vi "BT Example 1 - Repeater.vi"() -> ()   [LabVIEW 2021]
uses:
  Support/Nodes/abs_Node/Status.ctl
  Blackboard/Blackboard.lvclass
  Support/Nodes/Decorators/Repeater/Support/Finish On - Type.ctl
  System/bt_System.lvclass
  Blackboard/Blackboard.lvclass/Blackboard.ctl
  Blackboard/Get Value Type/Get I32.vi
  Blackboard/Support/Index Group.vi
  Blackboard/Support/Index Tags.vi
  <vilib>/TSA/Omni-Bus/Local Bus/Support/I32/Local Bus_I32.lvclass
  C:/Program Files (x86)/National Instruments/LabVIEW 2021/vi.lib/TSA/Abstract Data Classes/Abs_Types/Value/Abs_Value.lvclass
  <vilib>/TSA/Abstract Data Classes/Abs_Types/I32 Integer/Abs_I32 Integer.lvclass
  <vilib>/TSA/Omni-Bus/Local Bus/Support/Initialise DVR's.vi
  <vilib>/TSA/Abstract Data Classes/Functions/Math/Support/Increment/I32/Method.vi
  <vilib>/TSA/Abstract Data Classes/Abs_Types/Value/Abs_Value.lvclass
  <vilib>/TSA/Abstract Data Classes/Abs_Types/Type/Abs_Type.lvclass
  <vilib>/TSA/Omni-Bus/Local Bus/Support/DBL/Local Bus_DBL.lvclass
  <vilib>/TSA/Omni-Bus/Local Bus/Support/SGL/Local Bus_SGL.lvclass
  <vilib>/TSA/Omni-Bus/Local Bus/Support/EXT/Local Bus_EXT.lvclass
  <vilib>/TSA/Omni-Bus/Local Bus/Support/Bool/Local Bus_Boolean.lvclass
  <vilib>/TSA/Omni-Bus/Local Bus/Support/STR/Local Bus_String.lvclass
  <vilib>/TSA/Omni-Bus/Local Bus/Support/Variant/Local Bus_Variant.lvclass
  <vilib>/TSA/Omni-Bus/Local Bus/Support/WFM/Local Bus_Waveform.lvclass
  <vilib>/TSA/Omni-Bus/Local Bus/Support/Time/Local Bus_Time.lvclass
  <vilib>/TSA/Omni-Bus/Local Bus/Support/U8/Local Bus_U8.lvclass
  <vilib>/TSA/Omni-Bus/Local Bus/Support/U16/Local Bus_U16.lvclass
  <vilib>/TSA/Omni-Bus/Local Bus/Support/U32/Local Bus_U32.lvclass
  <vilib>/TSA/Omni-Bus/Local Bus/Support/U64/Local Bus_U64.lvclass
  <vilib>/TSA/Omni-Bus/Local Bus/Support/I8/Local Bus_I8.lvclass
  <vilib>/TSA/Omni-Bus/Local Bus/Support/I16/Local Bus_I16.lvclass
  <vilib>/TSA/Omni-Bus/Local Bus/Support/I64/Local Bus_I64.lvclass
  <vilib>/TSA/Omni-Bus/Local Bus/Support/CSGL/Local Bus_CSGL.lvclass
  <vilib>/TSA/Omni-Bus/Local Bus/Support/CDBL/Local Bus_CDBL.lvclass
  <vilib>/TSA/Omni-Bus/Local Bus/Support/CEXT/Local Bus_CEXT.lvclass
  <vilib>/TSA/Abstract Data Classes/Abs_Types/I32 Integer/Static Read.vi
  BT.lvlib
  Support/Nodes/Decorators/Repeater/bt_Repeater.lvclass
  <vilib>/TSA/Abstract Data Classes/Functions/Math/Support/Increment/I32/Increment_I32.lvclass
  Support/Nodes/abs_Node/bt_Node.lvclass
panel:
  out "Status":T1
  out "Count":i32
  in  "stop":bool
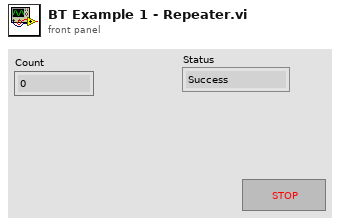
[diagram p1: front panel]
types:
  T1 = typedef "BT.lvlib/bt_Node.lvclass/Status.ctl" = enum16{"Success", "Failure", "Running"}
  T2 = typedef "BT.lvlib/bt_Repeater.lvclass/Finish On - Type.ctl" = enum16{"Success", "Failure", "Never"}
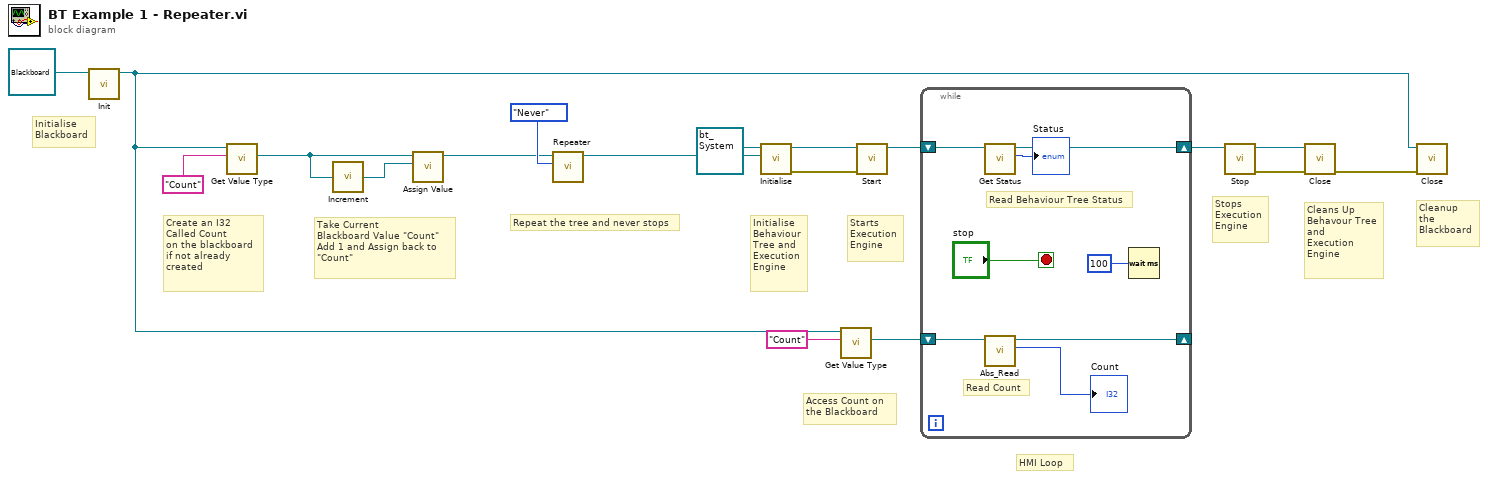
[diagram p0: block diagram]
diagram:
  # "Access Count on\nthe Blackboard"
  # "Create an I32\nCalled Count\non the blackboard\nif not already\ncreated"
  # "Initialise\nBlackboard"
  # "Cleanup\nthe\nBlackboard"
  # "Cleans Up\nBehavour Tree\nand\nExecution\nEngine"
  # "Initialise\nBehaviour\nTree and\nExecution\nEngine"
  # "Stops\nExecution\nEngine"
  # "Starts\nExecution\nEngine"
  # "HMI Loop"
  # "Repeat the tree and never stops"
  # "Take Current\nBlackboard Value \"Count\"\nAdd 1 and Assign back to \n\"Count\""
  n1 = call-dynamic "Init.vi"("bt_Blackboard in"=refnum<class "Blackboard.lvclass"> refnum) -> ("bt_Blackboard out"=w9:refnum<class "Blackboard.lvclass">)  [unwired: 9 in, 1 out]
  n2 = call-poly "Get Value Type.vi"("Tag"="Count", "Blackboard in"=w9) -> ("Value"=w8:refnum<class "Abs_I32 Integer.lvclass">)  [unwired: 6 in, 3 out]
  n3 = call-poly <vilib>:"Increment.vi"("Value"=w8) -> ("Result"=w11:refnum<class "Abs_I32 Integer.lvclass">)  [unwired: 4 in]
  n4 = call "Assign Value.vi"("Assigned Value"=w11, "Value"=w8) -> ("Node Out"=w1:refnum<class "bt_Node.lvclass">)  [unwired: 9 in]
  n5 = call "Repeater.vi"("Finish On"=Finish_On_-_Type."Never", "Node In"=w1) -> ("Node Out"=w3:refnum<class "bt_Node.lvclass">)  [unwired: 9 in]
  n6 = call "Initialise.vi"("Behaviour Tree"=w3, "bt_System in"=refnum<class "bt_System.lvclass"> refnum) -> ("error out"=w4:errorcluster, "bt_System out"=w5:refnum<class "bt_System.lvclass">)  [unwired: 8 in]
  n7 = call-poly "Get Value Type.vi"("Tag"="Count", "Blackboard in"=w9) -> ("Value"=w12:refnum<class "Abs_I32 Integer.lvclass">)  [unwired: 6 in, 3 out]
  n8 = call "Start.vi"("error in (no error)"=w4, "bt_System in"=w5) -> ("bt_System out"=w18:refnum<class "bt_System.lvclass">)  [unwired: 8 in, 1 out]
  n9 = while {
    shift-right: [w21] -> w17
    shift-left: w18 -> [w22]
    shift-right: [w25] -> _
    shift-left: w12 -> [w26]
    stop <- "stop" stop-if-true
    # "Read Behaviour Tree Status"
    # "Read Count"
    n10 = call "Get Status.vi"("bt_System in"=w22) -> ("Status"=→"Status":T1, "bt_System out"=w21:refnum<class "bt_System.lvclass">)  [unwired: 8 in, 1 out]
    n11 = call-poly <vilib>:"Abs_Read.vi"("Abs_I32 Integer in"=w26) -> ("Value"=→"Count":i32, "Abs_I32 Integer out"=w25:refnum<class "Abs_I32 Integer.lvclass">)  [unwired: 8 in, 1 out]
    n12 = Wait (ms)(milliseconds to wait=u32 100) -> ()  [unwired: 1 out]
  }
  n13 = call "Stop.vi"("bt_System in"=w17) -> ("error out"=w6:errorcluster, "bt_System out"=w7:refnum<class "bt_System.lvclass">)  [unwired: 9 in]
  n14 = call-dynamic "Close.vi"("error in (no error)"=w6, "bt_System in"=w7) -> ("error out"=w16:errorcluster)  [unwired: 8 in, 1 out]
  n15 = call-dynamic "Close.vi"("error in (no error)"=w16, "bt_Blackboard in"=w9) -> ()  [unwired: 8 in, 2 out]
